vi "Array STM fix.vi"(1 "Input array":dbl[][](array[numeric])) -> (0 "Output Array":dbl[][](array[numeric]))   [LabVIEW 2017]
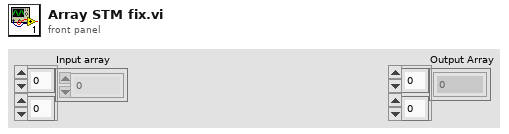
[diagram p1: front panel]
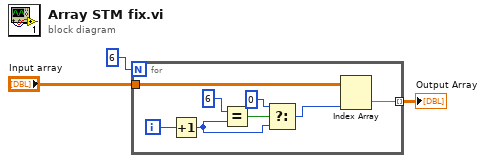
[diagram p0: block diagram]
diagram:
  n1 = for {
    N: 6 -> [_]
    tunnel: "Input array" -> [w10]
    tunnel: [w9] -> w2 mode=indexing
    i -> [w11]
    n2 = Increment(x=w11) -> (x+1=w4:i32)
    n3 = Equal?(x=6 ("y"), y=w4) -> (x = y?=w8:bool)
    n4 = Select(t=0, s=w8, f=w4) -> (s? t:f=w5:i32)
    n5 = Index Array(array=w10, index (col)=w5) -> (element=w9:dbl[])  [unwired: 1 in]
  }
  "Output Array" <- w2
